vi "Define Channel Count.vi"(8 "error in":errorcluster, 11 "module in":refnum<class "Module.lvclass">) -> (0 "error out":errorcluster, 3 "module out":refnum<class "Module.lvclass">)   [LabVIEW 2019, in "Scan Engine Scripting.lvlib" / "Module.lvclass"]
uses:
  Module.lvclass
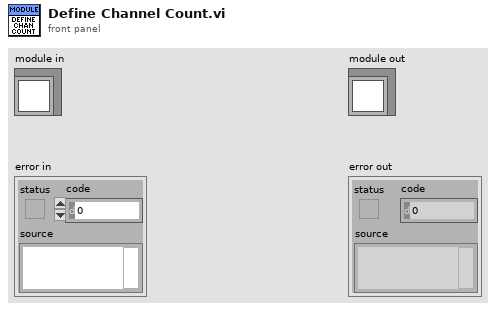
[diagram p1: front panel]
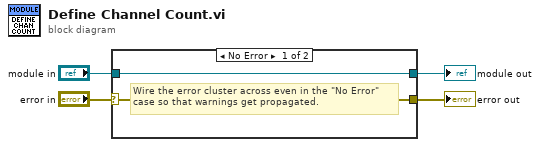
[diagram p0: block diagram]
diagram:
  n1 = case shown="No Error" "error in" {
    selector: "error in" -> [w5 w8]
    tunnel: [w5 w8] -> w3
    tunnel: [w6 w7] -> w1
    tunnel: "module in" -> [w6 w7]
    frame No Error {
      # "Wire the error cluster across even in the \"No Error\"\ncase so that warnings get propagated."
    }
    frame Error {
    }
  }
  "error out" <- w3
  "module out" <- w1
